vi "svl_Integration [frequency] Units.vi"(0 "spectrum":dbl[](array[numeric]) format="%.2f", 1 "f0":dbl format="%.2f", 2 "df [Hz]":dbl format="%.2f", 4 "spectrum info in":T2={"channel name"="", "description"="", "x-axis units"=0, "spectral info"={"spectrum type"=enum."Power [Magnitude^2]", "linear/dB"=enum."linear", "window"=0, "window size"=0, "FFT size"=0}, "engineering units"=0, "custom label"="", "dB reference [EU]"=0.0, "peak units"=enum."rms", "weighting filter"=0, "spectral density?"=FALSE, "unit label"="", "spectrum skewed?"=FALSE, "complimentary spectrum units"=enum."none"} {"x-axis units" items=["Time (s)"=0, "Frequency-CB (Hz)"=1, "Frequency-CPB (Hz)"=1248, "Frequency-Arbitrary (Hz)"=2357, "Quefrency (s)"=2, "Revolutions (rev)"=3, "Order"=4, "Speed (RPM)"=11, "Speed (rad/s)"=21, "Index"=65535]; "weighting filter" items=["Linear", "A-weighting", "B-weighting", "C-weighting", "ITU-R 468-4", "Dolby", "CCITT", "C-message", "Wb", "Wc", "Wd", "We", "Wf", "Wh", "Wj", "Wk", "Wm", "AES17 20 kHz lowpass", "AES17 40 kHz lowpass", "AES17 20 kHz highpass", "AES17 40 kHz highpass"]; "dB reference [EU]" format="%.2f"; "engineering units" items=["custom..."=0, "V"=1, "A"=21, "C"=30, "pC"=31, "s"=32, "-"=29, "Pa"=2, "N"=20, "g"=3, "m/s^2"=4, "m/s"=5, "m"=6, "mm/s"=12, "mm"=13, "micron/s"=14, "micron"=15, "in/s^2"=7, "in/s"=8, "in"=9, "mil/s"=10, "mil"=11, "rad/s^2"=16, "rad/s"=17, "rad"=18, "deg/s^2"=26, "deg/s"=27, "deg"=28, "RPM"=22, "cycle/s^2"=23, "Hz"=24, "cycle"=25, "strain"=19]; "spectral info"."window" items=["None "=0, "Hanning"=1, "Hamming"=2, "Blackman-Harris"=3, "Exact Blackman"=4, "Blackman"=5, "Flat Top"=6, "4 Term B-Harris "=7, "7 Term B-Harris"=8, "Low Sidelobe"=9, "Force - Exponential"=10, "Gaussian"=62]}, 5 "error in":errorcluster, 6 "integration type":T1(ring)=enum."double integration", 8 "desired base units for length":i32(ring) items=["no change"=-1, "m"=0, "mm"=2, "microns"=3, "in"=1, "mils"=5], 10 "automatically convert peak units":bool=TRUE) -> (14 "spectrum":dbl[](array[numeric]) format="%.2f", 15 "unit label":string, 18 "spectrum info out":T2={"channel name"="", "description"="", "x-axis units"=0, "spectral info"={"spectrum type"=enum."Power [Magnitude^2]", "linear/dB"=enum."linear", "window"=0, "window size"=0, "FFT size"=0}, "engineering units"=0, "custom label"="", "dB reference [EU]"=0.0, "peak units"=enum."rms", "weighting filter"=0, "spectral density?"=FALSE, "unit label"="", "spectrum skewed?"=FALSE, "complimentary spectrum units"=enum."none"} {"x-axis units" items=["Time (s)"=0, "Frequency-CB (Hz)"=1, "Frequency-CPB (Hz)"=1248, "Frequency-Arbitrary (Hz)"=2357, "Quefrency (s)"=2, "Revolutions (rev)"=3, "Order"=4, "Speed (RPM)"=11, "Speed (rad/s)"=21, "Index"=65535]; "weighting filter" items=["Linear", "A-weighting", "B-weighting", "C-weighting", "ITU-R 468-4", "Dolby", "CCITT", "C-message", "Wb", "Wc", "Wd", "We", "Wf", "Wh", "Wj", "Wk", "Wm", "AES17 20 kHz lowpass", "AES17 40 kHz lowpass", "AES17 20 kHz highpass", "AES17 40 kHz highpass"]; "dB reference [EU]" format="%.2f"; "engineering units" items=["custom..."=0, "V"=1, "A"=21, "C"=30, "pC"=31, "s"=32, "-"=29, "Pa"=2, "N"=20, "g"=3, "m/s^2"=4, "m/s"=5, "m"=6, "mm/s"=12, "mm"=13, "micron/s"=14, "micron"=15, "in/s^2"=7, "in/s"=8, "in"=9, "mil/s"=10, "mil"=11, "rad/s^2"=16, "rad/s"=17, "rad"=18, "deg/s^2"=26, "deg/s"=27, "deg"=28, "RPM"=22, "cycle/s^2"=23, "Hz"=24, "cycle"=25, "strain"=19]; "spectral info"."window" items=["None "=0, "Hanning"=1, "Hamming"=2, "Blackman-Harris"=3, "Exact Blackman"=4, "Blackman"=5, "Flat Top"=6, "4 Term B-Harris "=7, "7 Term B-Harris"=8, "Low Sidelobe"=9, "Force - Exponential"=10, "Gaussian"=62]}, 19 "error out":errorcluster)   [LabVIEW 2017, in "SoundVib_Integration.lvlib"]
uses:
  <vilib>/addons/Sound and Vibration/svt_Integration/SoundVib_Integration.lvlib
  <vilib>/addons/_NISVFA/_Shared subVIs/Controls/svc_Spectrum Info.ctl
  <vilib>/addons/_NISVFA/_Shared subVIs/Controls/svc_X-Axis Units.ctl
  <vilib>/addons/_NISVFA/_Shared subVIs/Controls/svc_Spectrum Type.ctl
  <vilib>/addons/_NISVFA/_Shared subVIs/Controls/svc_Engineering Units Text Ring.ctl
  <vilib>/addons/_NISVFA/_Shared subVIs/Controls/svc_Weighting Filter Text Ring.ctl
  <vilib>/addons/_NISVFA/_Shared subVIs/Controls/svc_Complimentary Spectrum Units.ctl
  <vilib>/addons/_NISVFA/_Spectrum Processing/subVIs/svfa_Peak to RMS to Peak2Peak.vi
  <vilib>/addons/_NISVFA/_Spectrum Processing/subVIs/svfa_Mag to Mag2.vi
  <vilib>/addons/_NISVFA/_Spectrum Processing/subVIs/svfa_Linear to dB.vi
  <vilib>/addons/_NISVFA/_Spectrum Processing/subVIs/svfa_dBrefA to dBrefB.vi
  <vilib>/addons/_NISVFA/_Spectrum Processing/subVIs/svfa_Spectrum to Spectral Density.vi
  <vilib>/addons/_NISVFA/_Shared subVIs/Common/svc_Get Weighting Enum and Labels.vi
  <vilib>/addons/_NISVFA/_Shared subVIs/Common/svc_Format Value (DBL).vi
  <vilib>/addons/_NISVFA/_Shared subVIs/Common/svc_Window Parameters.vi
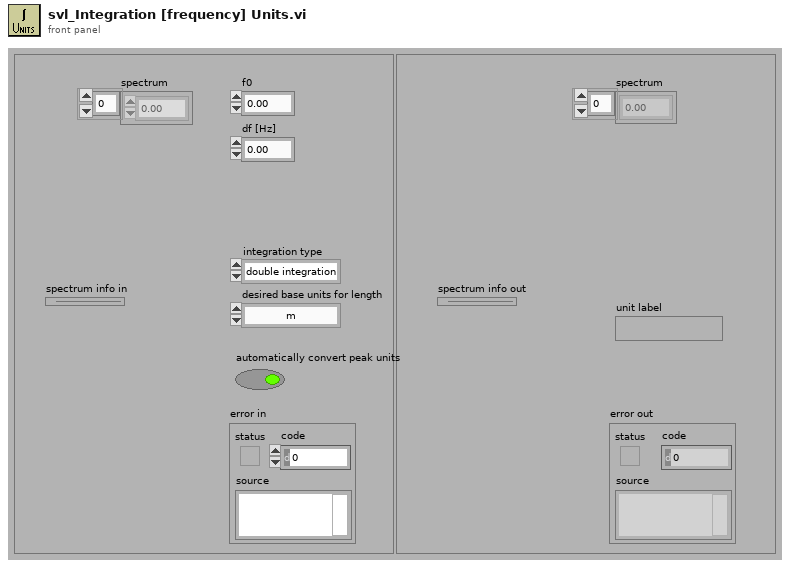
[diagram p1: front panel]
types:
  T1 = enum16{"single integration", "double integration"}
  T2 = typedef "svc_Spectrum Info.ctl" = cluster{"channel name":string, "description":string, "x-axis units":T3, "spectral info":cluster{"spectrum type":T4, "linear/dB":enum16{"linear", "dB"}, "window":u16, "window size":i32, "FFT size":i32}, "engineering units":T5, "custom label":string, "dB reference [EU]":dbl, "peak units":enum16{"rms", "peak", "peak-peak"}, "weighting filter":T6, "spectral density?":bool, "unit label":string, "spectrum skewed?":bool, "complimentary spectrum units":T7}
  T3 = typedef "svc_X-Axis Units.ctl" = u16
  T4 = typedef "svc_Spectrum Type.ctl" = enum16{"FFT Spectrum [complex]", "Amplitude [Magnitude]", "Power [Magnitude^2]", "Cross Spectrum [complex]", "Frequency Response [Complex]"}
  T5 = typedef "svc_Engineering Units Text Ring.ctl" = u16
  T6 = typedef "svc_Weighting Filter Text Ring.ctl" = u16
  T7 = typedef "svc_Complimentary Spectrum Units.ctl" = enum16{"none", "radians", "degrees", "cycles", "imaginary"}
  T8 = cluster{"linear/dB":enum16{"no change", "linear", "dB"}, "dB reference (0: no change)":dbl, "power/magnitude":enum16{"no change", "power", "magnitude"}, "view":enum16{"no change", "rms", "peak", "peak-peak"}}
  T9 = enum16{"no change", "spectrum", "spectral density"}
  T10 = enum16{"custom...", "V", "Pa", "g", "m/s^2", "m/s", "m", "in/s^2", "in/s", "in", "mil/s", "mil", "mm/s", "mm", "micron/s", "micron", "rad/s^2", "rad/s", "rad", "strain", "N", "A", "rpm", "cycle/s^2", "Hz", "cycle", "deg/s^2", "deg/s", "deg", "Undefined", "C", "pC"}
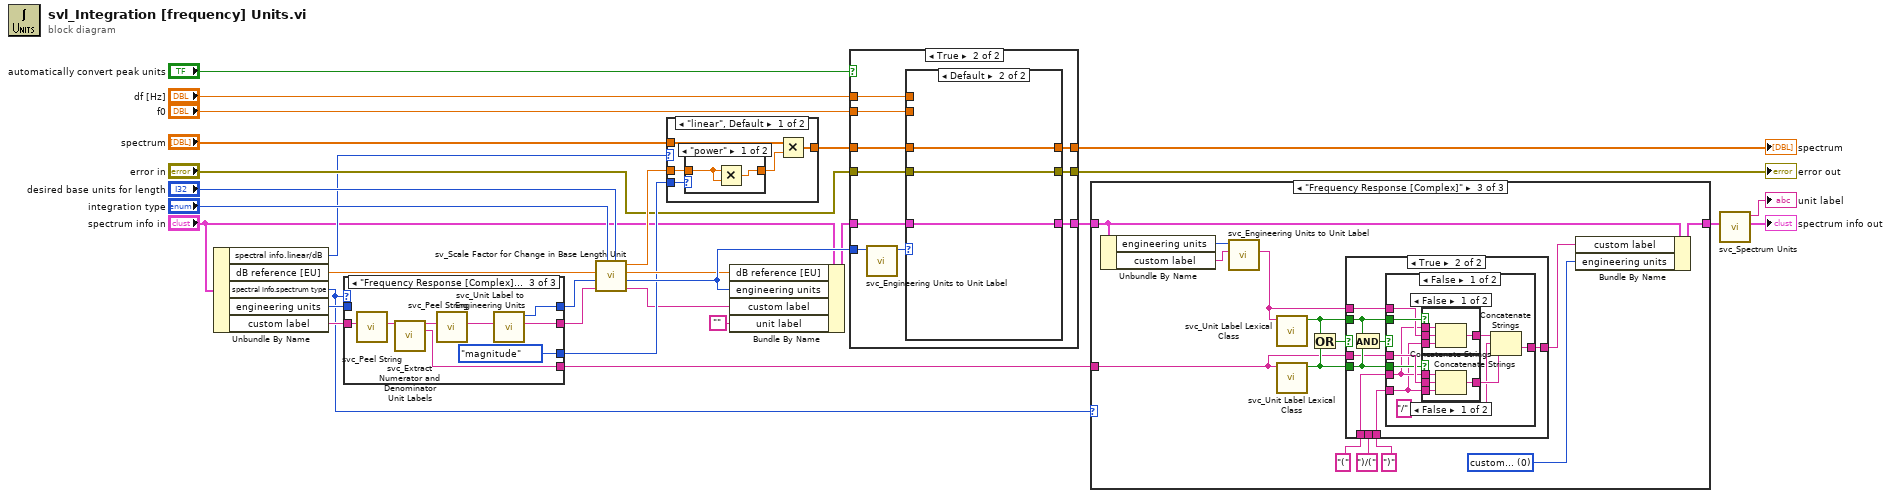
[diagram p0: block diagram]
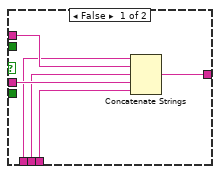
[diagram p6: hidden frame]
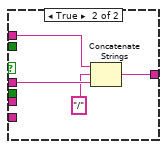
[diagram p9: hidden frame]
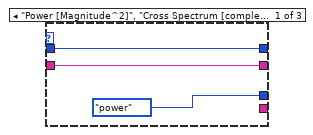
[diagram p10: hidden frame]
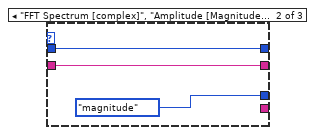
[diagram p11: hidden frame]
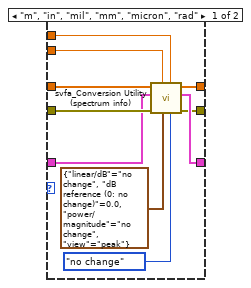
[diagram p13: hidden frame]
diagram:
  n1 = Unbundle By Name("spectrum info in") -> ("spectral info.linear/dB"=w4:enum16{"linear", "dB"}, "dB reference [EU]"=w16:dbl, "spectral info.spectrum type"=w19:T4, "engineering units"=w22:T5, "custom label"=w21:string)
  n2 = case shown="\"Frequency Response [Complex]\"" w19 {
    tunnel: [enum16{"power", "magnitude"}."power" ("power/magnitude") enum16{"power", "magnitude"}."magnitude" ("power/magnitude") enum16{"power", "magnitude"}."magnitude" ("power/magnitude")] -> w9
    tunnel: [w32 w35 w38] -> w15
    tunnel: w22 -> [w32 w35 _]
    tunnel: [w31 w34 w37] -> w14
    tunnel: w21 -> [w31 w34 w43]
    tunnel: [_ _ w41] -> w20
    frame "Power [Magnitude^2]", "Cross Spectrum [complex]", Default {
    }
    frame "FFT Spectrum [complex]", "Amplitude [Magnitude]" {
    }
    frame "Frequency Response [Complex]" {
      n3 = call <vilib>:"svc_Peel String.vi"("string"=w43) -> ("peeled string"=w40:string)  [unwired: 10 in]
      n4 = call <vilib>:"svc_Extract Numerator and Denominator Unit Labels.vi"("unit label"=w40) -> ("numerator unit label"=w42:string, "denominator unit label"=w41:string)  [unwired: 13 in]
      n5 = call <vilib>:"svc_Peel String.vi"("string"=w42) -> ("peeled string"=w39:string)  [unwired: 10 in]
      n6 = call <vilib>:"svc_Unit Label to Engineering Units.vi"("unit label"=w39) -> ("unit label out"=w37:string, "engineering units"=w38:T5)  [unwired: 9 in]
    }
  }
  n7 = call <vilib>:"sv_Scale Factor for Change in Base Length Unit.vi"("desired base units for length"="desired base units for length", "integration type"="integration type", "custom label in"=w14, "engineering units in"=w15, "dB reference [EU] in"=w16) -> ("custom label out"=w1:string, "engineering units out"=w13:T5, "dB reference [EU] out"=w12:dbl, "units scale factor"=w7:dbl)  [unwired: 3 in]
  n8 = case shown="\"linear\", Default" w4 {
    tunnel: "spectrum" -> [w49 w53]
    tunnel: w9 -> [w48 _]
    tunnel: w7 -> [w47 _]
    tunnel: [w45 w53] -> w6
    frame "linear", Default {
      n9 = case shown="\"power\"" w48 {
        tunnel: [w50 w52] -> w46
        tunnel: w47 -> [w51 w52]
        frame "power" {
          n10 = Multiply(x=w51, y=w51) -> (x*y=w50:dbl)
        }
        frame "magnitude", Default {
        }
      }
      n11 = Multiply(x=w49, y=w46) -> (x*y=w45:dbl[])
    }
    frame "dB" {
    }
  }
  n12 = Bundle By Name(cluster="spectrum info in", "dB reference [EU]"=w12, "engineering units"=w13, "custom label"=w1, "unit label"="") -> (w2:T2)
  n13 = case shown="True" "automatically convert peak units" {
    tunnel: w2 -> [w56 w63]
    tunnel: [w55 w66] -> w30
    tunnel: [w56 w65] -> w18
    tunnel: "error in" -> [w55 w64]
    tunnel: w13 -> [_ w61]
    tunnel: w6 -> [w54 w60]
    tunnel: [w54 w59] -> w23
    tunnel: "df [Hz]" -> [_ w58]
    tunnel: "f0" -> [_ w57]
    frame False {
    }
    frame True {
      n14 = call <vilib>:"svc_Engineering Units to Unit Label.vi"("engineering units"=w61) -> ("engineering units enum"=w62:T10)  [unwired: 9 in, 1 out]
      n15 = case shown="Default" w62 {
        tunnel: w63 -> [w75 w77]
        tunnel: [w72 w79] -> w66
        tunnel: [w74 w77] -> w65
        tunnel: w64 -> [w76 w79]
        tunnel: w60 -> [w73 w78]
        tunnel: [w71 w78] -> w59
        tunnel: w58 -> [w70 _]
        tunnel: w57 -> [w69 _]
        frame "m", "in", "mil", "mm", "micron", "rad" {
          n16 = call <vilib>:"svfa_Conversion Utility (spectrum info).vi"("spectral density desired"=T9."no change", "dx"=w70, "desired scaling"=T8 {"linear/dB"=enum."no change", "dB reference (0: no change)"=0.0, "power/magnitude"=enum."no change", "view"=enum."peak"}, "x0"=w69, "error in (no error)"=w76, "spectrum info in"=w75, "input signal"=w73) -> ("error out"=w72:errorcluster, "spectrum info out"=w74:T2, "converted signal"=w71:dbl[])  [unwired: 2 in]
        }
        frame Default {
        }
      }
    }
  }
  "spectrum" <- w23
  "error out" <- w30
  n17 = case shown="\"Frequency Response [Complex]\"" w19 {
    tunnel: w20 -> [_ _ w83]
    tunnel: w18 -> [w80 w81 w95]
    tunnel: [w80 w81 w94] -> w17
    frame "Power [Magnitude^2]", "Cross Spectrum [complex]", Default {
    }
    frame "FFT Spectrum [complex]", "Amplitude [Magnitude]" {
    }
    frame "Frequency Response [Complex]" {
      w93 = T5 0 items=["custom..."=0, "V"=1, "A"=21, "Pa"=2, "N"=20, "g"=3, "m/s^2"=4, "m/s"=5, "m"=6, "mm/s"=12, "mm"=13, "micron/s"=14, "micron"=15, "in/s^2"=7, "in/s"=8, "in"=9, "mil/s"=10, "mil"=11, "rad/s^2"=16, "rad/s"=17, "rad"=18, "deg/s^2"=26, "deg/s"=27, "deg"=28, "RPM"=22, "cycle/s^2"=23, "Hz"=24, "cycle"=25, "strain"=19] ("engineering units")
      n18 = Unbundle By Name(w95) -> ("engineering units"=w92:T5, "custom label"=w91:string)
      n19 = call <vilib>:"svc_Engineering Units to Unit Label.vi"("custom label"=w91, "engineering units"=w92) -> ("unit label"=w84:string)  [unwired: 8 in, 1 out]
      n20 = call <vilib>:"svc_Unit Label Lexical Class.vi"("unit label"=w84) -> ("letters only?"=w86:bool)  [unwired: 6 in]
      n21 = call <vilib>:"svc_Unit Label Lexical Class.vi"("unit label"=w83) -> ("letters only?"=w85:bool)  [unwired: 6 in]
      n22 = Or(x=w86, y=w85) -> (x .or. y?=w87:bool)
      n23 = case shown="True" w87 {
        tunnel: w84 -> [w101 w106]
        tunnel: w83 -> [w100 w105]
        tunnel: [w99 w104] -> w82
        tunnel: ")" ("Substring") -> [w98 w102]
        tunnel: ")/(" ("Substring") -> [w97 _]
        tunnel: "(" ("Substring") -> [w96 w103]
        tunnel: w86 -> [_ w108]
        tunnel: w85 -> [_ w109]
        frame False {
          n24 = Concatenate Strings(w96, w101, w97, w100, w98) -> (w99:string)
        }
        frame True {
          n25 = And(x=w108, y=w109) -> (x .and. y?=w107:bool)
          n26 = case shown="False" w107 {
            tunnel: w109 -> [w116 _]
            tunnel: w108 -> [w119 _]
            tunnel: w106 -> [w118 w133]
            tunnel: w105 -> [w117 w132]
            tunnel: [w111 w131] -> w104
            tunnel: w103 -> [w115 _]
            tunnel: w102 -> [w114 _]
            frame False {
              n27 = case shown="False" w119 {
                tunnel: w118 -> [w128 w129]
                tunnel: [w125 w129] -> w113
                tunnel: w115 -> [w127 _]
                tunnel: w114 -> [w126 _]
                frame False {
                  n28 = Concatenate Strings(w127, w128, w126) -> (w125:string)
                }
                frame True {
                }
              }
              n29 = case shown="False" w116 {
                tunnel: w117 -> [w123 w124]
                tunnel: [w122 w124] -> w112
                tunnel: w115 -> [w121 _]
                tunnel: w114 -> [w120 _]
                frame False {
                  n30 = Concatenate Strings(w121, w123, w120) -> (w122:string)
                }
                frame True {
                }
              }
              n31 = Concatenate Strings(w113, "/" ("Substring"), w112) -> (w111:string)
            }
            frame True {
              n32 = Concatenate Strings(w133, "/" ("string"), w132) -> (w131:string)
            }
          }
        }
      }
      n33 = Bundle By Name(cluster=w95, "custom label"=w82, "engineering units"=w93) -> (w94:T2)
    }
  }
  n34 = call <vilib>:"svc_Spectrum Units.vi"("spectrum info in"=w17) -> ("spectrum info out"=→"spectrum info out":T2, "unit label"=→"unit label":string)  [unwired: 3 in, 2 out]
